vi "MCB2300 Write Digital AI Conflict ProjectAttrValidator.vi"(5 "Ctl Refnum":refnum<vi>, 7 "IO Name (original)":string, 9 "IO Channel Number":i32(ring) items=["0", "1", "2", "3", "4", "5", "6", "7", "8", "9", "10", "11", "12", "13", "14", "15", "16", "17", "18", "19", "20", "21", "22", "23", "24", "25", "26", "27", "28", "29", "30", "31", "32", "33", "34", "35", "36", "37", "38", "39", "40", "41", "42", "43", "44", "45", "46", "47", "48", "49", "50", "51", "52", "53", "54", "55", "56", "57", "58", "59", "60", "61", "62", "63", "64", "65", "66", "67", "68", "69", "70", "71", "72", "73", "74", "75", "76", "77", "78", "79", "80", "81", "82", "83", "84", "85", "86", "87", "88", "89", "90", "91", "92", "93", "94", "95", "96", "97", "98", "99", "100", "101", "102", "103", "104", "105", "106", "107", "108", "109", "110", "111", "112", "113", "114", "115", "116", "117", "118", "119", "120", "121", "122", "123", "124", "125", "126", "127", "128", "129", "130", "131", "132", "133", "134", "135", "136", ""], 11 "Project Attributes":T1 {"Programmable Pin Connections" items=["AI0 uses pin P0.23. You cannot use AI0 and pin P0.23 in the same project.", "AI1 uses pin P0.24. You cannot use AI1 and pin P0.24 in the same project. ", "AI2 uses pin P0.25. You cannot use AI2 and pin P0.25 in the same project.", "AI3 uses pin P0.26. You cannot use AI3 and pin P0.26 in the same project.", "AI4 uses pin P1.30. You cannot use AI4 and pin P1.30 in the same project.", "AI5 uses pin P1.31. You cannot use AI5 and pin P1.31 in the same project.", "AI6 uses pin P0.12. You cannot use AI6 and pin P0.12 in the same project.", "AI7 uses pin P0.13. You cannot use AI7 and pin P0.13 in the same project."]}) -> (3 "Valid?":bool)   [LabVIEW 2011]
uses:
  <vilib>/Embedded/ARM/MCB2300/MCB2300_AI_Conflicts_PrjAttr.ctl
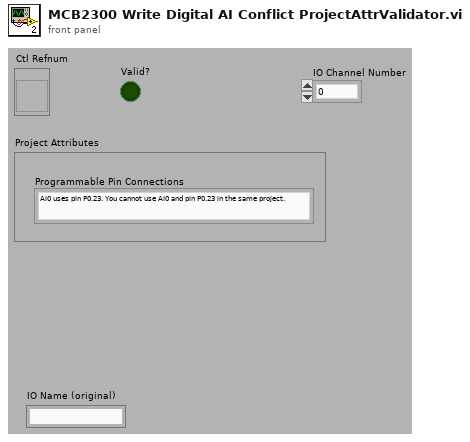
[diagram p1: front panel]
types:
  T1 = typedef "MCB2300_AI_Conflicts_PrjAttr.ctl" = cluster{"Programmable Pin Connections":u16}
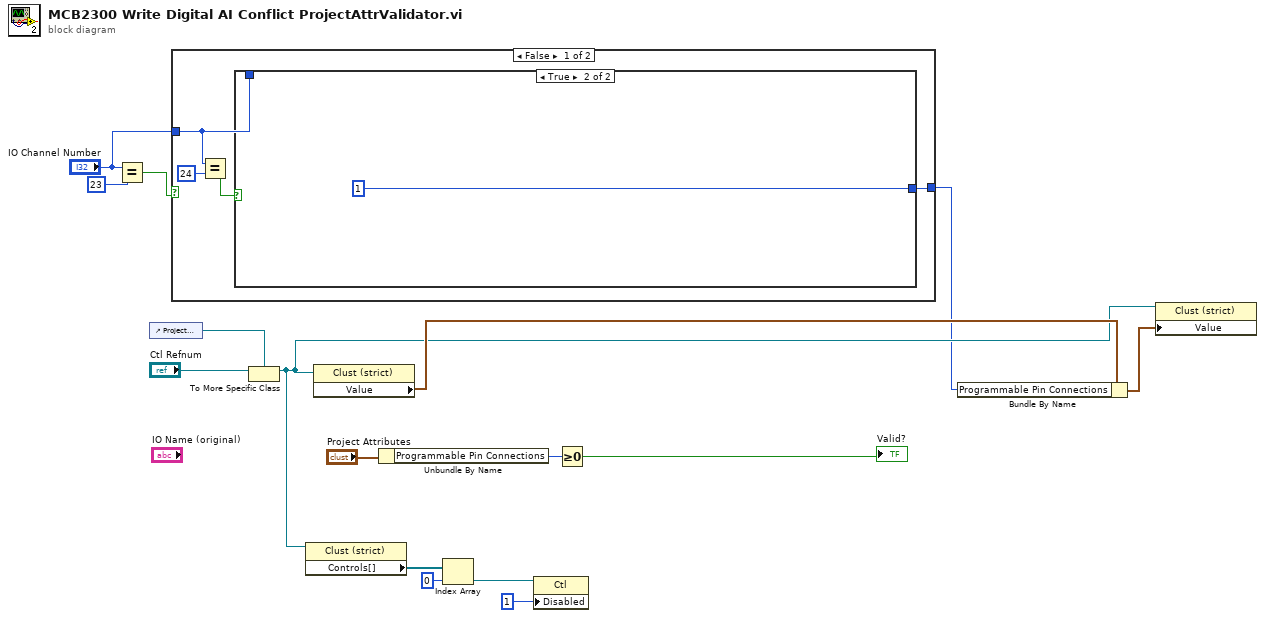
[diagram p0: block diagram]
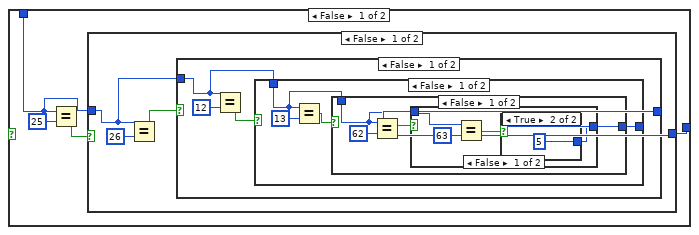
[diagram p2: hidden frame]
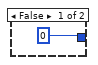
[diagram p3: hidden frame]
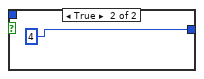
[diagram p4: hidden frame]
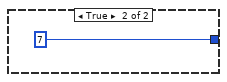
[diagram p5: hidden frame]
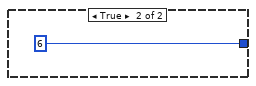
[diagram p6: hidden frame]
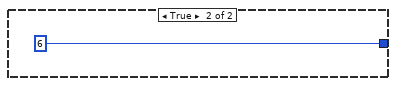
[diagram p7: hidden frame]
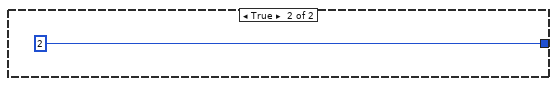
[diagram p8: hidden frame]
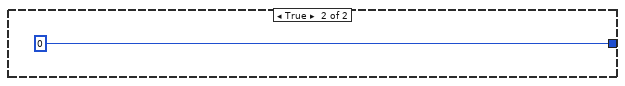
[diagram p9: hidden frame]
diagram:
  n1 = Equal?(x="IO Channel Number", y=23) -> (x = y?=w2:bool)
  n2 = control-ref of="Project Attributes"() -> (w15:refnum<vi>)
  n3 = case shown="False" w2 {
    tunnel: [w18 0] -> w3
    tunnel: "IO Channel Number" -> [w17 _]
    frame False {
      n4 = Equal?(x=w17, y=24) -> (x = y?=w19:bool)
      n5 = case shown="True" w19 {
        tunnel: [w22 1] -> w18
        tunnel: w17 -> [w21 _]
        frame False {
          n6 = Equal?(x=w21, y=25) -> (x = y?=w23:bool)
          n7 = case shown="False" w23 {
            tunnel: [w26 2] -> w22
            tunnel: w21 -> [w25 _]
            frame False {
              n8 = Equal?(x=w25, y=26) -> (x = y?=w27:bool)
              n9 = case shown="False" w27 {
                tunnel: [w30 6] -> w26
                tunnel: w25 -> [w29 _]
                frame False {
                  n10 = Equal?(x=w29, y=12) -> (x = y?=w31:bool)
                  n11 = case shown="False" w31 {
                    tunnel: [w34 6] -> w30
                    tunnel: w29 -> [w33 _]
                    frame False {
                      n12 = Equal?(x=w33, y=13) -> (x = y?=w35:bool)
                      n13 = case shown="False" w35 {
                        tunnel: [w38 7] -> w34
                        tunnel: w33 -> [w37 _]
                        frame False {
                          n14 = Equal?(x=w37, y=62) -> (x = y?=w39:bool)
                          n15 = case shown="False" w39 {
                            tunnel: [w41 4] -> w38
                            tunnel: w37 -> [w43 _]
                            frame False {
                              n16 = Equal?(x=w43, y=63) -> (x = y?=w42:bool)
                              n17 = case shown="True" w42 {
                                tunnel: [0 5] -> w41
                                frame False {
                                }
                                frame True {
                                }
                              }
                            }
                            frame True {
                            }
                          }
                        }
                        frame True {
                        }
                      }
                    }
                    frame True {
                    }
                  }
                }
                frame True {
                }
              }
            }
            frame True {
            }
          }
        }
        frame True {
        }
      }
    }
    frame True {
    }
  }
  n18 = To More Specific Class(target class=w15, reference="Ctl Refnum") -> (specific class reference=w5:refnum<vi>)  [unwired: 1 in, 1 out]
  n19 = property class="Clust (strict)"(reference=w5) -> ("Controls[]"=w12:refnum<vi>[])  [unwired: 1 in, 2 out]
  n20 = property class="Clust (strict)"(reference=w5) -> ("Value"=w14:cluster{"Programmable Pin Connections":u16})  [unwired: 1 in, 2 out]
  n21 = Unbundle By Name("Project Attributes") -> ("Programmable Pin Connections"=w7:u16)
  n22 = Index Array(array=w12, index=0) -> (element=w10:refnum<vi>)
  n23 = property class="Ctl"(reference=w10, "Disabled"=u8 1) -> ()  [unwired: 1 in, 2 out]
  n24 = Greater Or Equal To 0?(x=w7) -> (x >= 0?=→"Valid?":bool)
  n25 = Bundle By Name(cluster=w14, "Programmable Pin Connections"=w3) -> (w13:cluster{"Programmable Pin Connections":u16})
  n26 = property class="Clust (strict)"(reference=w5, "Value"=w13) -> ()  [unwired: 1 in, 2 out]
